vi "Numeric Check Output Result.vi"(9 "Output Value in":cluster{"Name":string, "Variant Data":variant}, 10 "Step Output in":T5, 11 "Execution in":refnum<data-value>) -> (2 "Measure Result out":T1, 3 "Execution out":refnum<data-value>)   [LabVIEW 2015, in "Execution.lvclass"]
uses:
  Execution.lvclass
  Step/STEP_OUTPUT.ctl
  Step/OUTPUT_DATA_TYPE.ctl
  OutputUI/OUTPUT_CHECK_TYPE.ctl
  Step/OUTPUT_VALUE_TYPE.ctl
  STEP_MEASURE_RESULT.ctl
  Step/STEP_STATUS.ctl
  <vilib>/Utility/error.llb/DialogType.ctl
  Get Limit Value Numeric.vi
  Step.lvclass
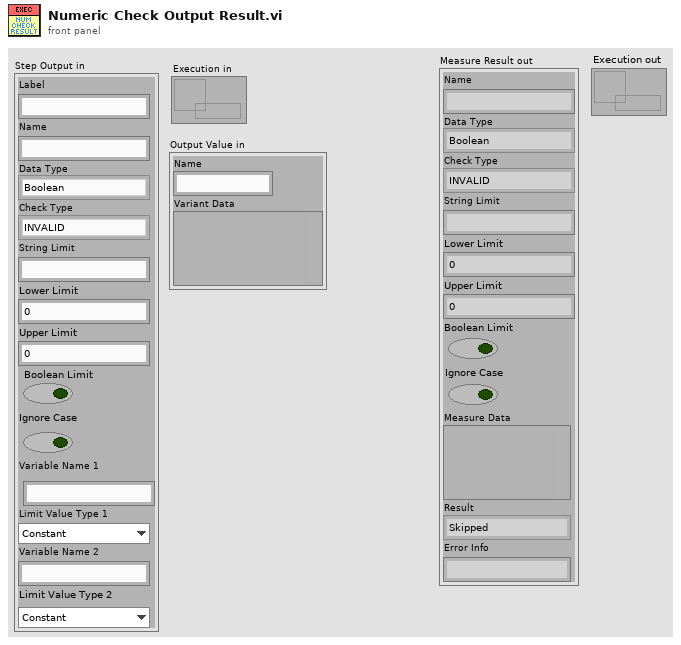
[diagram p1: front panel]
types:
  T1 = typedef "Execution.lvclass/STEP_MEASURE_RESULT.ctl" = cluster{"Name":string, "Data Type":T2, "Check Type":T3, "String Limit":string, "Lower Limit":dbl, "Upper Limit":dbl, "Boolean Limit":bool, "Ignore Case":bool, "Measure Data":variant, "Result":T4, "Error Info":string}
  T2 = typedef "Step.lvclass/OUTPUT_DATA_TYPE.ctl" = enum16{"Boolean", "String", "Numeric", "Other"}
  T3 = typedef "Step.lvclass/OUTPUT_CHECK_TYPE.ctl" = enum16{"INVALID", "DO_NOT_CHECK", "RECORD", "VARIABLE", "EQUAL", "NOT_EQUAL", "STR_CONTAINS", "STR_START_WITH", "STR_END_WITH", "STR_REGEX_MATCH", "NUM_GT", "NUM_LT", "NUM_GE", "NUM_LE", "NUM_RANGE", "NUM_RANGE_BDY"}
  T4 = typedef "Step.lvclass/STEP_STATUS.ctl" = enum16{"Skipped", "Done", "Passed", "Failed", "Error"}
  T5 = typedef "Step.lvclass/STEP_OUTPUT.ctl" = cluster{"Label":string, "Name":string, "Data Type":T2, "Check Type":T3, "String Limit":string, "Lower Limit":dbl, "Upper Limit":dbl, "Boolean Limit":bool, "Ignore Case":bool, "Variable Name 1":string, "Limit Value Type 1":T6, "Variable Name 2":string, "Limit Value Type 2":T6}
  T6 = typedef "Step.lvclass/OUTPUT_VALUE_TYPE.ctl" = enum16{"Constant", "Variable"}
  T7 = typedef "DialogType.ctl" = u16
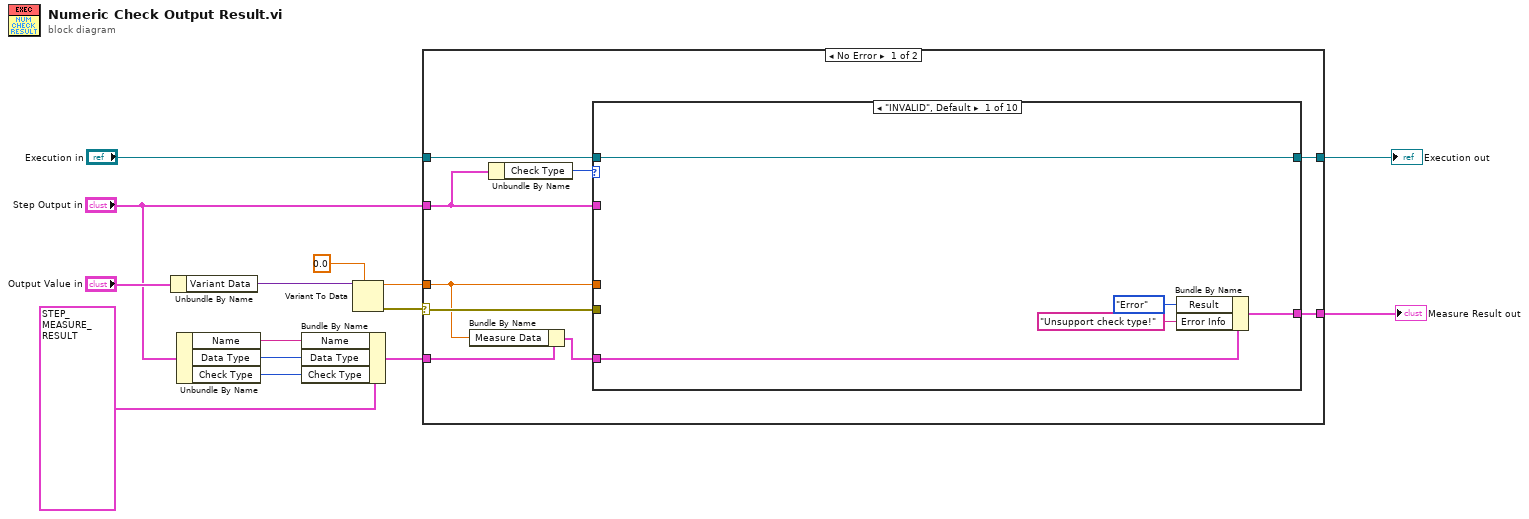
[diagram p0: block diagram]
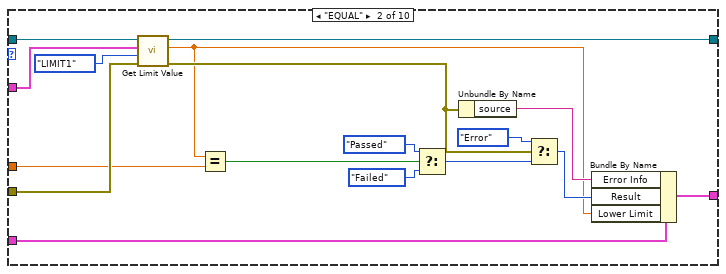
[diagram p2: hidden frame]
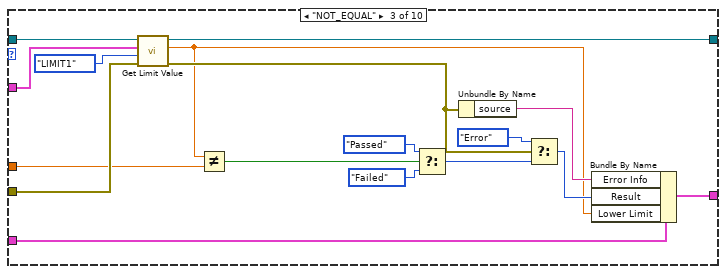
[diagram p3: hidden frame]
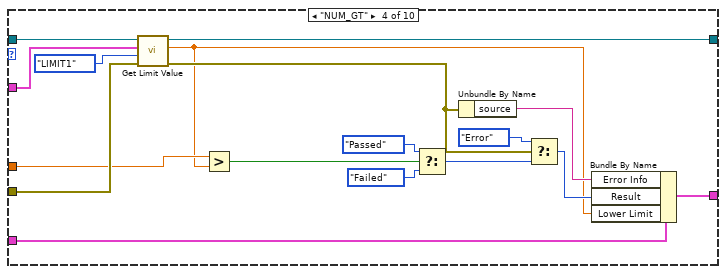
[diagram p4: hidden frame]
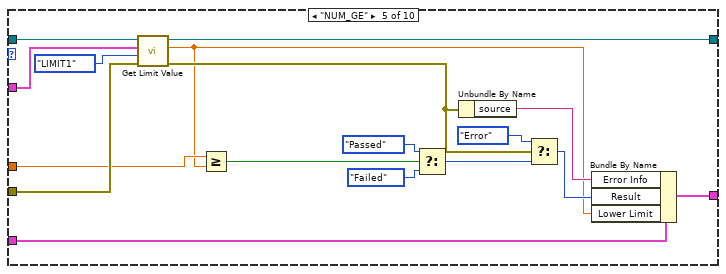
[diagram p5: hidden frame]
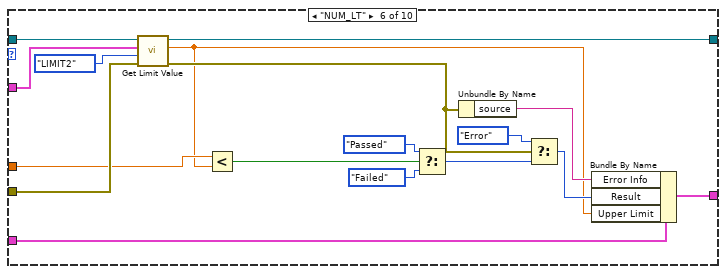
[diagram p6: hidden frame]
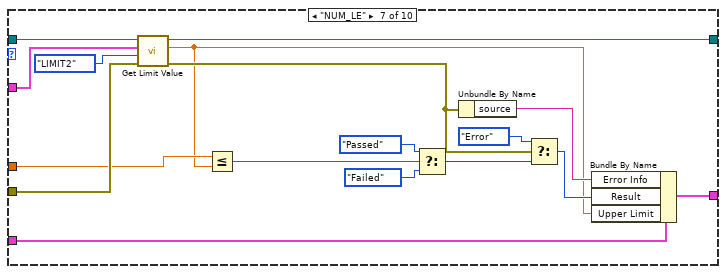
[diagram p7: hidden frame]
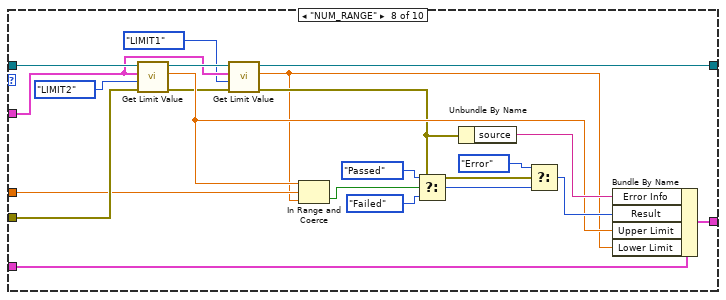
[diagram p8: hidden frame]
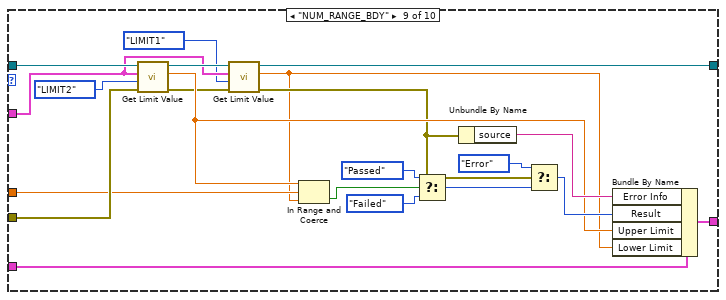
[diagram p9: hidden frame]
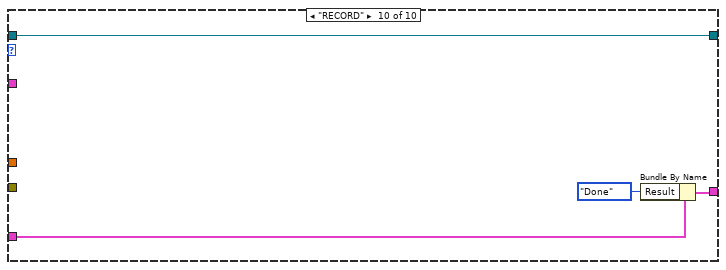
[diagram p10: hidden frame]
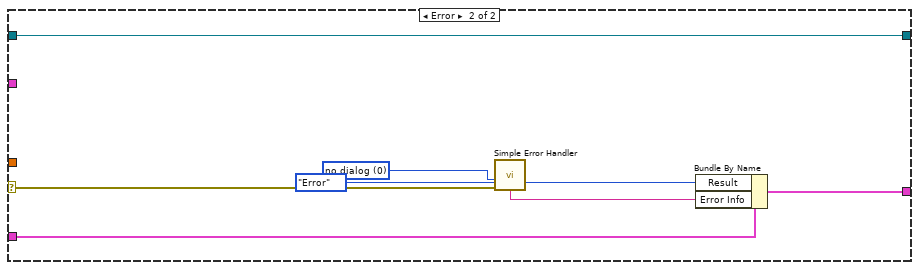
[diagram p11: hidden frame]
diagram:
  n1 = Unbundle By Name("Output Value in") -> ("Variant Data"=w12:variant)
  n2 = Unbundle By Name("Step Output in") -> ("Name"=w5:string, "Data Type"=w4:T2, "Check Type"=w3:T3)
  n3 = Bundle By Name(cluster=T1 {"Name"="", "Data Type"=enum."Boolean", "Check Type"=enum."INVALID", "String Limit"="", "Lower Limit"=0.0, "Upper Limit"=0.0, "Boolean Limit"=FALSE, "Ignore Case"=FALSE, "Measure Data"=variant, "Result"=enum."Skipped", "Error Info"=""} ("Measure Result"), "Name"=w5, "Data Type"=w4, "Check Type"=w3) -> (w2:T1)
  n4 = Variant To Data(type=0.0, Variant=w12) -> (data=w10:dbl, error out=w14:errorcluster)  [unwired: 1 in]
  n5 = case shown="No Error" w14 {
    selector: w14 -> [w20 w182]
    tunnel: "Step Output in" -> [w23 _]
    tunnel: w10 -> [w18 _]
    tunnel: "Execution in" -> [w22 w181]
    tunnel: [w21 w181] -> w8
    tunnel: w2 -> [w19 w180]
    tunnel: [w16 w177] -> w1
    frame No Error {
      n6 = Bundle By Name(cluster=w19, "Measure Data"=w18) -> (w17:T1)
      n7 = Unbundle By Name(w23) -> ("Check Type"=w15:T3)
      n8 = case shown="\"INVALID\", Default" w15 {
        tunnel: w23 -> [_ w32 w49 w66 w83 w100 w117 w136 w157 _]
        tunnel: w18 -> [_ w29 w46 w64 w81 w98 w115 w140 w161 _]
        tunnel: w22 -> [w28 w37 w54 w71 w88 w105 w122 w143 w164 w173]
        tunnel: [w28 w36 w53 w70 w87 w104 w121 w137 w158 w173] -> w21
        tunnel: w20 -> [_ w35 w52 w69 w86 w103 w120 w142 w163 _]
        tunnel: w17 -> [w27 w41 w58 w75 w92 w109 w126 w147 w168 w176]
        tunnel: [w24 w38 w55 w72 w89 w106 w123 w144 w165 w175] -> w16
        frame "INVALID", Default {
          n9 = Bundle By Name(cluster=w27, "Result"=STEP_STATUS."Error" ("Status"), "Error Info"="Unsupport check type!") -> (w24:T1)
        }
        frame "EQUAL" {
          n10 = call-poly "Get Limit Value.vi"("error in (no error)"=w35, "Limit"=enum16{"LIMIT1", "LIMIT2"}."LIMIT1", "Step Output in"=w32, "Execution in"=w37) -> ("error out"=w33:errorcluster, "Limit Value"=w30:dbl, "Execution out"=w36:refnum<data-value>)  [unwired: 5 in]
          n11 = Equal?(x=w30, y=w29) -> (x = y?=w31:bool)
          n12 = Select(t=STEP_STATUS."Passed" ("Status"), s=w31, f=STEP_STATUS."Failed" ("Status")) -> (s? t:f=w43:T4)
          n13 = Unbundle By Name(w33) -> ("source"=w39:string)
          n14 = Select(t=STEP_STATUS."Error" ("Status"), s=w33, f=w43) -> (s? t:f=w40:T4)
          n15 = Bundle By Name(cluster=w41, "Error Info"=w39, "Result"=w40, "Lower Limit"=w30) -> (w38:T1)
        }
        frame "NOT_EQUAL" {
          n16 = call-poly "Get Limit Value.vi"("error in (no error)"=w52, "Limit"=enum16{"LIMIT1", "LIMIT2"}."LIMIT1", "Step Output in"=w49, "Execution in"=w54) -> ("error out"=w50:errorcluster, "Limit Value"=w47:dbl, "Execution out"=w53:refnum<data-value>)  [unwired: 5 in]
          n17 = Not Equal?(x=w47, y=w46) -> (x != y?=w48:bool)
          n18 = Select(t=STEP_STATUS."Passed" ("Status"), s=w48, f=STEP_STATUS."Failed" ("Status")) -> (s? t:f=w60:T4)
          n19 = Unbundle By Name(w50) -> ("source"=w56:string)
          n20 = Select(t=STEP_STATUS."Error" ("Status"), s=w50, f=w60) -> (s? t:f=w57:T4)
          n21 = Bundle By Name(cluster=w58, "Error Info"=w56, "Result"=w57, "Lower Limit"=w47) -> (w55:T1)
        }
        frame "NUM_GT" {
          n22 = call-poly "Get Limit Value.vi"("error in (no error)"=w69, "Limit"=enum16{"LIMIT1", "LIMIT2"}."LIMIT1", "Step Output in"=w66, "Execution in"=w71) -> ("error out"=w67:errorcluster, "Limit Value"=w63:dbl, "Execution out"=w70:refnum<data-value>)  [unwired: 5 in]
          n23 = Greater?(x=w64, y=w63) -> (0:w65:bool)
          n24 = Select(t=STEP_STATUS."Passed" ("Status"), s=w65, f=STEP_STATUS."Failed" ("Status")) -> (s? t:f=w77:T4)
          n25 = Unbundle By Name(w67) -> ("source"=w73:string)
          n26 = Select(t=STEP_STATUS."Error" ("Status"), s=w67, f=w77) -> (s? t:f=w74:T4)
          n27 = Bundle By Name(cluster=w75, "Error Info"=w73, "Result"=w74, "Lower Limit"=w63) -> (w72:T1)
        }
        frame "NUM_GE" {
          n28 = call-poly "Get Limit Value.vi"("error in (no error)"=w86, "Limit"=enum16{"LIMIT1", "LIMIT2"}."LIMIT1", "Step Output in"=w83, "Execution in"=w88) -> ("error out"=w84:errorcluster, "Limit Value"=w80:dbl, "Execution out"=w87:refnum<data-value>)  [unwired: 5 in]
          n29 = Greater Or Equal?(x=w81, y=w80) -> (x >= y?=w82:bool)
          n30 = Select(t=STEP_STATUS."Passed" ("Status"), s=w82, f=STEP_STATUS."Failed" ("Status")) -> (s? t:f=w94:T4)
          n31 = Unbundle By Name(w84) -> ("source"=w90:string)
          n32 = Select(t=STEP_STATUS."Error" ("Status"), s=w84, f=w94) -> (s? t:f=w91:T4)
          n33 = Bundle By Name(cluster=w92, "Error Info"=w90, "Result"=w91, "Lower Limit"=w80) -> (w89:T1)
        }
        frame "NUM_LT" {
          n34 = call-poly "Get Limit Value.vi"("error in (no error)"=w103, "Limit"=enum16{"LIMIT1", "LIMIT2"}."LIMIT2", "Step Output in"=w100, "Execution in"=w105) -> ("error out"=w101:errorcluster, "Limit Value"=w97:dbl, "Execution out"=w104:refnum<data-value>)  [unwired: 5 in]
          n35 = Less?(x=w98, y=w97) -> (x < y?=w99:bool)
          n36 = Select(t=STEP_STATUS."Passed" ("Status"), s=w99, f=STEP_STATUS."Failed" ("Status")) -> (s? t:f=w111:T4)
          n37 = Unbundle By Name(w101) -> ("source"=w107:string)
          n38 = Select(t=STEP_STATUS."Error" ("Status"), s=w101, f=w111) -> (s? t:f=w108:T4)
          n39 = Bundle By Name(cluster=w109, "Error Info"=w107, "Result"=w108, "Upper Limit"=w97) -> (w106:T1)
        }
        frame "NUM_LE" {
          n40 = call-poly "Get Limit Value.vi"("error in (no error)"=w120, "Limit"=enum16{"LIMIT1", "LIMIT2"}."LIMIT2", "Step Output in"=w117, "Execution in"=w122) -> ("error out"=w118:errorcluster, "Limit Value"=w114:dbl, "Execution out"=w121:refnum<data-value>)  [unwired: 5 in]
          n41 = Less Or Equal?(x=w115, y=w114) -> (x <= y?=w116:bool)
          n42 = Select(t=STEP_STATUS."Passed" ("Status"), s=w116, f=STEP_STATUS."Failed" ("Status")) -> (s? t:f=w128:T4)
          n43 = Unbundle By Name(w118) -> ("source"=w124:string)
          n44 = Select(t=STEP_STATUS."Error" ("Status"), s=w118, f=w128) -> (s? t:f=w125:T4)
          n45 = Bundle By Name(cluster=w126, "Error Info"=w124, "Result"=w125, "Upper Limit"=w114) -> (w123:T1)
        }
        frame "NUM_RANGE" {
          n46 = call-poly "Get Limit Value.vi"("error in (no error)"=w142, "Limit"=enum16{"LIMIT1", "LIMIT2"}."LIMIT2", "Step Output in"=w136, "Execution in"=w143) -> ("error out"=w134:errorcluster, "Limit Value"=w139:dbl, "Execution out"=w138:refnum<data-value>)  [unwired: 5 in]
          n47 = call-poly "Get Limit Value.vi"("error in (no error)"=w134, "Limit"=enum16{"LIMIT1", "LIMIT2"}."LIMIT1", "Step Output in"=w136, "Execution in"=w138) -> ("error out"=w133:errorcluster, "Limit Value"=w132:dbl, "Execution out"=w137:refnum<data-value>)  [unwired: 5 in]
          n48 = In Range and Coerce(upper limit=w139, x=w140, lower limit=w132) -> (In Range?=w131:bool)  [unwired: 1 out]
          n49 = Select(t=STEP_STATUS."Passed" ("Status"), s=w131, f=STEP_STATUS."Failed" ("Status")) -> (s? t:f=w149:T4)
          n50 = Unbundle By Name(w133) -> ("source"=w145:string)
          n51 = Select(t=STEP_STATUS."Error" ("Status"), s=w133, f=w149) -> (s? t:f=w146:T4)
          n52 = Bundle By Name(cluster=w147, "Error Info"=w145, "Result"=w146, "Upper Limit"=w139, "Lower Limit"=w132) -> (w144:T1)
        }
        frame "NUM_RANGE_BDY" {
          n53 = call-poly "Get Limit Value.vi"("error in (no error)"=w163, "Limit"=enum16{"LIMIT1", "LIMIT2"}."LIMIT2", "Step Output in"=w157, "Execution in"=w164) -> ("error out"=w155:errorcluster, "Limit Value"=w160:dbl, "Execution out"=w159:refnum<data-value>)  [unwired: 5 in]
          n54 = call-poly "Get Limit Value.vi"("error in (no error)"=w155, "Limit"=enum16{"LIMIT1", "LIMIT2"}."LIMIT1", "Step Output in"=w157, "Execution in"=w159) -> ("error out"=w154:errorcluster, "Limit Value"=w153:dbl, "Execution out"=w158:refnum<data-value>)  [unwired: 5 in]
          n55 = In Range and Coerce(upper limit=w160, x=w161, lower limit=w153) -> (In Range?=w152:bool)  [unwired: 1 out]
          n56 = Select(t=STEP_STATUS."Passed" ("Status"), s=w152, f=STEP_STATUS."Failed" ("Status")) -> (s? t:f=w170:T4)
          n57 = Unbundle By Name(w154) -> ("source"=w166:string)
          n58 = Select(t=STEP_STATUS."Error" ("Status"), s=w154, f=w170) -> (s? t:f=w167:T4)
          n59 = Bundle By Name(cluster=w168, "Error Info"=w166, "Result"=w167, "Upper Limit"=w160, "Lower Limit"=w153) -> (w165:T1)
        }
        frame "RECORD" {
          n60 = Bundle By Name(cluster=w176, "Result"=STEP_STATUS."Done") -> (w175:T1)
        }
      }
    }
    frame Error {
      w183 = T7 0 items=["no dialog", "OK message", "continue or stop message", "OK message + warnings", "continue/stop + warnings"] ("type of dialog (OK msg:1)")
      n61 = call <vilib>:"Simple Error Handler.vi"("type of dialog (OK msg:1)"=w183, "error in (no error)"=w182) -> ("message"=w179:string)  [unwired: 3 in, 4 out]
      n62 = Bundle By Name(cluster=w180, "Result"=STEP_STATUS."Error" ("Status"), "Error Info"=w179) -> (w177:T1)
    }
  }
  "Execution out" <- w8
  "Measure Result out" <- w1
